vi "PDF.vi"() -> ()   [LabVIEW 2014]
panel:
  out "PDF项目":string
  out "PDF焊接固化料车条码":string
  out "PDF当前状态":string
  out "PDF焊接上料车条码":string
  out "PDF焊接工位生产信息":string[][](table)
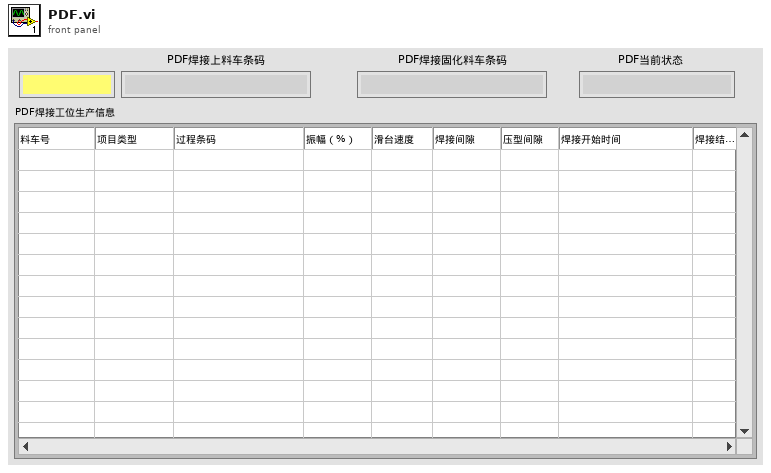
[diagram p1: front panel]
types:
  T1 = cluster{"PDF焊接工位生产信息":refnum<vi>, "PDF焊接上料车条码":refnum<vi>, "PDF当前状态":refnum<vi>, "PDF焊接固化料车条码":refnum<vi>, "PDF项目":refnum<vi>}
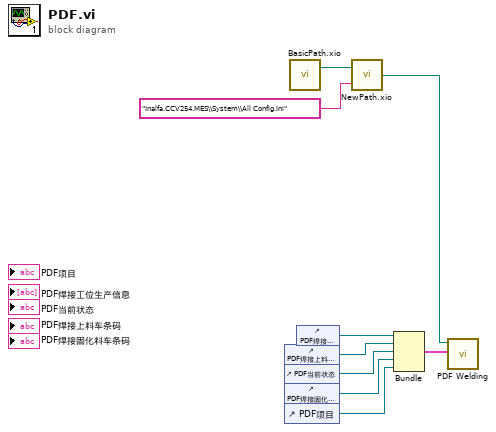
[diagram p0: block diagram]
diagram:
  n1 = control-ref of="PDF焊接上料车条码"() -> (w6:refnum<vi>)
  n2 = control-ref of="PDF当前状态"() -> (w5:refnum<vi>)
  n3 = control-ref of="PDF焊接固化料车条码"() -> (w3:refnum<vi>)
  n4 = control-ref of="PDF项目"() -> (w2:refnum<vi>)
  n5 = call "BasicPath.xio.vi"() -> ("stripped path"=w8:path)  [unwired: 1 in, 1 out]
  n6 = control-ref of="PDF焊接工位生产信息"() -> (w7:refnum<vi>)
  n7 = call "NewPath.xio.vi"("Append path"="Inalfa.CCV254.MES\\System\\All Config.ini", "Basic path"=w8) -> ("New path"=w1:path)
  n8 = Bundle("PDF焊接工位生产信息"=w7, "PDF焊接上料车条码"=w6, "PDF当前状态"=w5, "PDF焊接固化料车条码"=w3, "PDF项目"=w2) -> (w4:T1)  [unwired: 1 in]
  n9 = call "PDF Welding.vi"("configuration file path"=w1, "PDF Welding msic inf"=w4) -> ()  [unwired: 4 in]
